vi "FTW-TestExecutiveGUI-FormatSequenceForDisplay.vi"(0 "Sequence":T1[](array[typedef]) {"Results"."Start Time" format="%<%Y-%m-%d %H:%M:%S%03u>T"; "Results"."Elapsed Time" format="%<%H:%M:%S%3u>t"; "Elapsed Time" format="%<%H:%M:%S%3u>t"}, 11 "error in":errorcluster) -> (4 "Table":string[][](array[string]), 15 "error out":errorcluster)   [LabVIEW 2015]
doc: "Can be used to interpret the following messages\n\nSequenceLoaded\nSequenceComplete\nStepChange"
uses:
  source/actor/TestExecutive/FTW-TestExecutive-Step.ctl
  source/actor/TestExecutive/FTW-TestExecutive-Step-State.ctl
  source/actor/TestExecutive/FTW-TestExecutive-Results.ctl
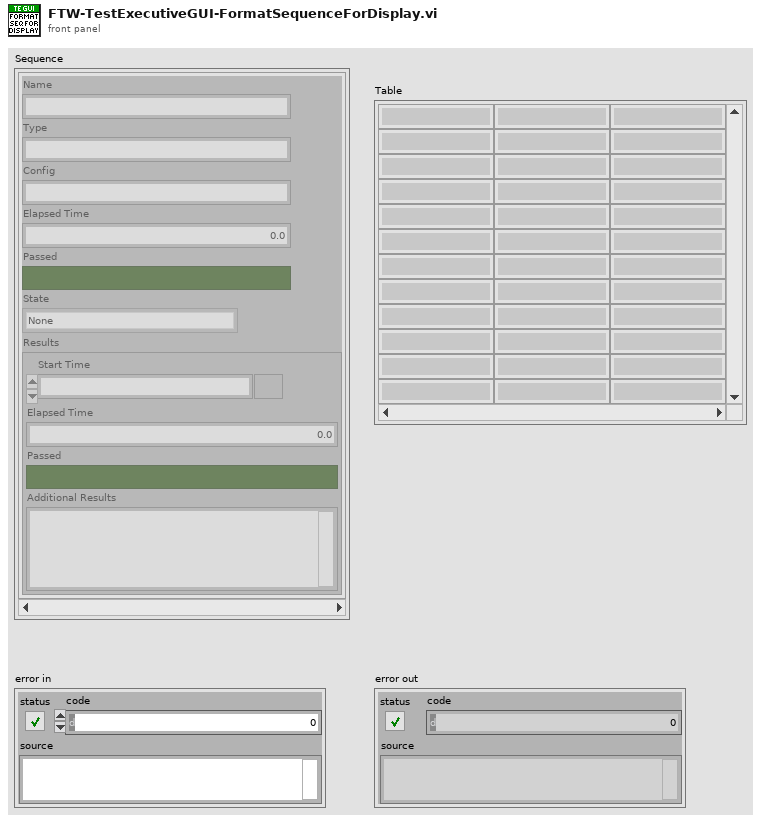
[diagram p1: front panel]
types:
  T1 = typedef "FTW-TestExecutive-Step.ctl" = cluster{"Name":string, "Type":string, "Config":string, "Elapsed Time":dbl, "Passed":bool, "State":T2, "Results":T3}
  T2 = typedef "FTW-TestExecutive-Step-State.ctl" = enum8{"None", "Failed", "Passed", "Timed out", "Aborted"}
  T3 = typedef "FTW-TestExecutive-Results.ctl" = cluster{"Start Time":timestamp, "Elapsed Time":dbl, "Passed":bool, "Additional Results":string}
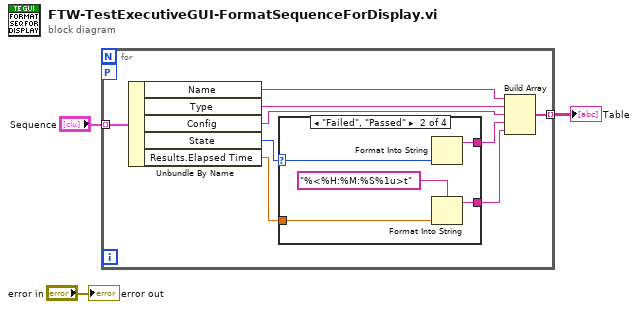
[diagram p0: block diagram]
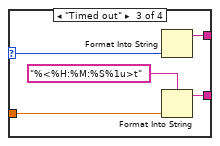
[diagram p3: hidden frame]
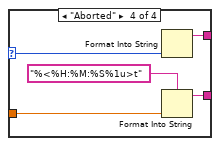
[diagram p4: hidden frame]
diagram:
  n1 = for {
    tunnel: "Sequence" -> [w12] mode=indexing
    tunnel: [w10] -> w1 mode=indexing
    workers-P: _ -> [_]
    n2 = Unbundle By Name(w12) -> ("Name"=w11:string, "Type"=w9:string, "Config"=w8:string, "State"=w5:T2, "Results.Elapsed Time"=w7:dbl)
    n3 = case shown="\"Failed\", \"Passed\"" w5 {
      selector: w5 -> [_ w13 w18 w23]
      tunnel: w7 -> [_ w17 w22 w27]
      tunnel: [_ w15 w20 w25] -> w6
      tunnel: [_ w14 w19 w24] -> w4
      frame "None" {
      }
      frame "Failed", "Passed" {
        n4 = Format Into String(w13) -> (resulting string=w14:string)  [unwired: 3 in, 1 out]
        n5 = Format Into String(format string="%<%H:%M:%S%1u>t", w17) -> (resulting string=w15:string)  [unwired: 2 in, 1 out]
      }
      frame "Timed out" {
        n6 = Format Into String(w18) -> (resulting string=w19:string)  [unwired: 3 in, 1 out]
        n7 = Format Into String(format string="%<%H:%M:%S%1u>t", w22) -> (resulting string=w20:string)  [unwired: 2 in, 1 out]
      }
      frame "Aborted" {
        n8 = Format Into String(w23) -> (resulting string=w24:string)  [unwired: 3 in, 1 out]
        n9 = Format Into String(format string="%<%H:%M:%S%1u>t", w27) -> (resulting string=w25:string)  [unwired: 2 in, 1 out]
      }
    }
    n10 = Build Array(w11, w9, w8, w4, w6) -> (w10:string[])
  }
  "Table" <- w1
  "error out" <- "error in"
